vi "StartTestSuite.vi"(8 "error in (no error)":errorcluster, 10 "TestSuite":refnum<class "TestSuite.lvclass">, 11 "ResultTreeListener in":refnum<class "ResultTreeListener.lvclass">) -> (0 "error out":errorcluster, 3 "ResultTreeListener out":refnum<class "ResultTreeListener.lvclass">)   [LabVIEW 2019, in "ResultTreeListener.lvclass"]
doc: "A test suite started."
uses:
  ResultTreeListener.lvclass
  TestSuite/TestSuite.lvclass
  ResultTreeListener.lvclass/ResultTreeListener.ctl
  ResultTree/ResultTree.lvclass
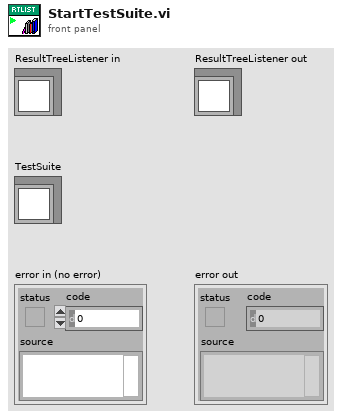
[diagram p1: front panel]
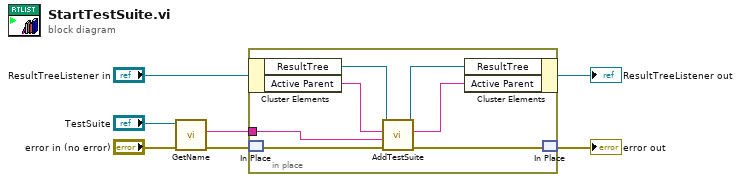
[diagram p0: block diagram]
diagram:
  n1 = call-dynamic "GetName.vi"("error in (no error)"="error in (no error)", "TestSuite in"="TestSuite") -> ("error out"=w2:errorcluster, "Name"=w7:string)  [unwired: 7 in, 1 out]
  n2 = in-place {
    in-place-border: w7 -> [w14]
    n3 = in-place-cluster #1("ResultTreeListener in") -> ("ResultTree"=w13:refnum<class "ResultTree.lvclass">, "Active Parent"=w8:string)
    n4 = in-place-match #2(w2) -> (w11:errorcluster)
    n5 = call "AddTestSuite.vi"("error in (no error)"=w11, "Name"=w14, "Parent Tag (\"\")"=w8, "ResultTree in"=w13) -> ("error out"=w10:errorcluster, "Tag Name"=w9:string, "ResultTree out"=w12:refnum<class "ResultTree.lvclass">)  [unwired: 5 in]
    n6 = in-place-cluster #1("ResultTree"=w12, "Active Parent"=w9) -> (→"ResultTreeListener out":refnum<class "ResultTreeListener.lvclass">)
    n7 = in-place-match #2(w10) -> (→"error out":errorcluster)
  }
